vi "FindPeak.vi"(1 "Input Array":dbl[](array[numeric])) -> (0 "Index of Peak":dbl)   [LabVIEW 2013]
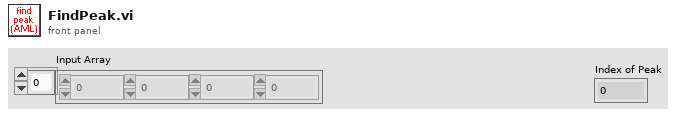
[diagram p1: front panel]
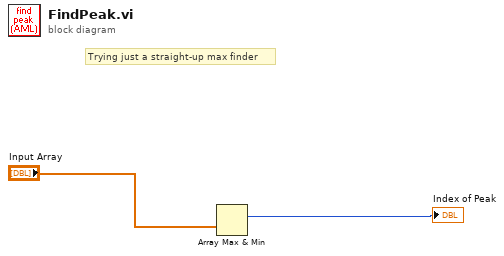
[diagram p0: block diagram]
diagram:
  # "Trying just a straight-up max finder"
  n1 = Array Max & Min(array="Input Array") -> (max index (indices)=→"Index of Peak":i32)  [unwired: 3 out]
